vi "Refresh Status Tree.vi"(6 "Show Metrics":bool, 7 "Tree Ref":refnum<vi>, 8 "error in (no error)":errorcluster, 11 "Debug GUI Module in":refnum<class "Debug GUI Module.lvclass">) -> (0 "error out":errorcluster, 3 "Debug GUI Module out":refnum<class "Debug GUI Module.lvclass">)   [LabVIEW 2020, in "VolatusGUI.lvlib" / "Debug GUI Module.lvclass"]
uses:
  Debug GUI Module.lvclass
  Volatus/StatusTreeValue/StatusTreeValue.lvclass
  Debug GUI Module.lvclass/Debug GUI Module.ctl
  lv-tree-tools/Tree Map/Tree Map/Tree Map.lvclass
  Volatus/MessageQ/MessageQ.lvclass
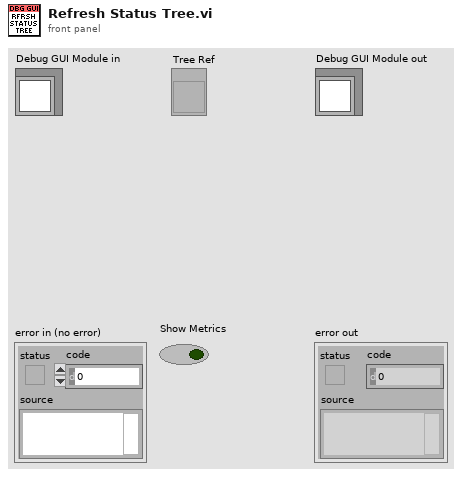
[diagram p1: front panel]
types:
  T1 = typedef "VolatusGUI.lvlib/Debug GUI Module.lvclass/Node Status.ctl" = cluster{"URL":string, "Status Tree":map{string[], T2}}
  T2 = typedef "Volatus.lvlib/Module Status.ctl" = cluster{"Hierarchy":string[], "State":T3, "Substatus":map{string, string}, "Metrics":map{string, dbl}}
  T3 = typedef "Volatus.lvlib/Module.lvclass/State.ctl" = enum16{"Unknown", "Launched", "Starting", "Running", "Stopping", "Stopped", "Error - Starting", "Error - Run", "Error - Stopping"}
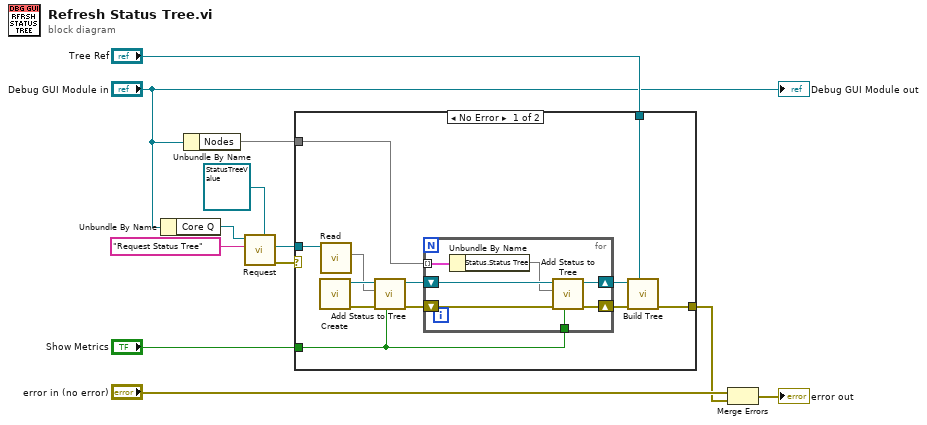
[diagram p0: block diagram]
diagram:
  n1 = Unbundle By Name("Debug GUI Module in") -> ("Core Q"=w10:refnum<class "MessageQ.lvclass">)
  n2 = Unbundle By Name("Debug GUI Module in") -> ("Nodes"=w2:map{string, T1})
  n3 = call "Request.vi"("Response Type (None)"=refnum<class "StatusTreeValue.lvclass"> refnum ("Volatus:StatusTreeValue.lvclass"), "ID"="Request Status Tree", "MessageQ in"=w10) -> ("error out"=w6:errorcluster, "Response"=w5:refnum<class "StatusTreeValue.lvclass">)  [unwired: 6 in, 1 out]
  n4 = case shown="No Error" w6 {
    selector: w6 -> [_ w32]
    tunnel: "Tree Ref" -> [w24 _]
    tunnel: w5 -> [w23 _]
    tunnel: [w22 w32] -> w4
    tunnel: w2 -> [w16 _]
    tunnel: "Show Metrics" -> [w13 _]
    frame No Error {
      n5 = call "Create.vi"() -> ("error out"=w20:errorcluster, "Tree Map out"=w21:refnum<class "Tree Map.lvclass">)  [unwired: 10 in]
      n6 = call "Read.vi"("StatusTreeValue in"=w23) -> ("Status Tree"=w19:map{string[], T2})  [unwired: 10 in]
      n7 = call "Add Status to Tree.vi"("Show Metrics"=w13, "error in"=w20, "Status Tree"=w19, "Tree Map in"=w21) -> ("error out"=w18:errorcluster, "Tree Map"=w17:refnum<class "Tree Map.lvclass">)  [unwired: 6 in]
      n8 = for {
        shift-right: [w26] -> w14
        shift-left: w18 -> [w30]
        shift-right: [w27] -> w15
        shift-left: w17 -> [w31]
        tunnel: w16 -> [w29] mode=indexing
        tunnel: w13 -> [w25]
        n9 = Unbundle By Name(w29) -> ("Status.Status Tree"=w28:map{string[], T2})
        n10 = call "Add Status to Tree.vi"("Show Metrics"=w25, "error in"=w30, "Status Tree"=w28, "Tree Map in"=w31) -> ("error out"=w26:errorcluster, "Tree Map"=w27:refnum<class "Tree Map.lvclass">)  [unwired: 6 in]
      }
      n11 = call "Build Tree.vi"("Tree"=w24, "error in (no error)"=w14, "Tree Map in"=w15) -> ("error out"=w22:errorcluster)  [unwired: 7 in, 1 out]
    }
    frame Error {
    }
  }
  n12 = Merge Errors("error in (no error)", w4) -> (→"error out":errorcluster)
  "Debug GUI Module out" <- "Debug GUI Module in"
